vi "alarmacu.vi"() -> ()   [LabVIEW 2011]
panel:
  out "Mensaje":string
  out "Alarma":bool
  in  "Numeric":dbl
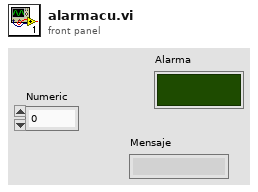
[diagram p1: front panel]
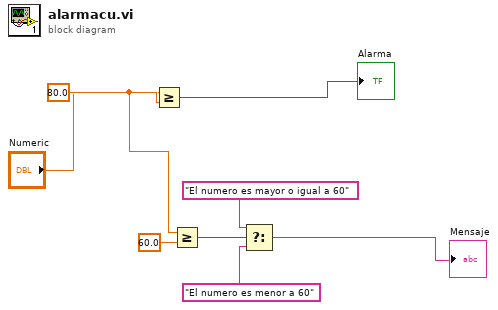
[diagram p0: block diagram]
diagram:
  n1 = Greater Or Equal?(x="Numeric", y=80.0 ("x")) -> (x >= y?=→"Alarma":bool)
  n2 = Greater Or Equal?(x="Numeric", y=60.0) -> (x >= y?=w6:bool)
  n3 = Select(t="El numero es mayor o igual a 60", s=w6, f="El numero es menor a 60") -> (s? t:f=→"Mensaje":string)
